vi "libpthread path.vi"(8 "error in (no error)":errorcluster) -> (0 "error out":errorcluster, 3 "path to libpthread":path)   [LabVIEW 2013, in "POSIX Threads.lvlib" / "POSIX Thread Object.lvclass"]
uses:
  POSIX Thread Object.lvclass
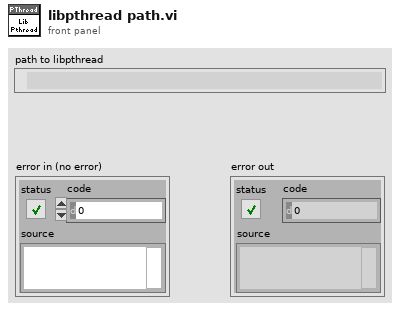
[diagram p1: front panel]
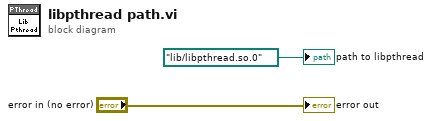
[diagram p0: block diagram]
diagram:
  "path to libpthread" <- path "/lib/libpthread.so.0" ("path to shared object")
  "error out" <- "error in (no error)"
